vi "Curtin_DAQ.vi"(11 "Settings":T1={"Name of test"="SoundCard--NI 01", "Date"=timestamp(0 s since 1904-01-01), "Location"="Home", "Template"="ScratchPad", "Soundcard"="OCTA-CAPTURE", "resolution"=32, "Sampling rate"=48000, "Ch1 Gain "=1.0, "Ch2 Gain"=1.0, "Sample time (s)"=0.3, "Pre-trigger (s)"=0.001, "Hammer Threshold"=10.0, "Positions"=7, "Taps/Position"=5, "Set Names"="H", "Freq resolution"=1.0, "Hammer cutoff"=0.025, "Mic cutoff"=0.25, "Double bounce "=10.0, "Hammer Cal"=1.0, "dB Offset"=0.0, "Accel Cal"=1.0, "Vibrometer Cal"=1.0, "Mic Cal"=1.0, "Output"=2, "Voltage Cal"=1.0, "Vibrometer Port"="ASRL27::INSTR", "Range"=10, "High Pass"=2, "Bandwidth"=10, "X Range"=[], "Y Range"=[], "dB Spread"=40.0, "Trigger"=0, "Ch_1"=1, "Ch_2"=1, "flip?"=FALSE, "60Hz"=FALSE, "Time offset"=0.0, "Piezo Cal"=1.0, "Default Notes"=""} {"Ch_2" min=1 step=1; "Ch_1" min=1 max=100 step=1; "Trigger" items=["Hammer (force)", "Self-tap", "Spacebar"]; "Bandwidth" items=["1 kHz"=1, "5 kHz"=5, "10 kHz"=10, "25 kHz"=25, "50 kHz"=50, "100 kHz"=100]; "High Pass" items=["Off", "13 Hz", "104 Hz"]; "Range" items=["10 mm/s"=1, "20 mm/s"=2, "50 mm/s"=5, "100 mm/s"=10, "200 mm/s"=20, "500 mm/s"=50, "1 m/s"=100, "2 m/s"=200]; "Output" items=["Accelerometer", "Speed (from acceleration)", "Microphone", "Vibrometer", "Piezo"]; "Voltage Cal" format="%#_13g"; "Ch2 Gain" format="%#_13g"; "Ch1 Gain" format="%#_13g"; "Double bounce" min=0.0; "Mic cutoff" min=0.0 format="%#_4g"; "Hammer cutoff" min=0.0 format="%#_4g"; "Freq resolution" min=0.0; "Pre-trigger (s)" format="%#_13g"; "Date" format="%<%H:%M\n%d/%m/%y>T"; "resolution" items=["16 bit"=16, "24 bit"=24, "32 bit"=32]; "Sampling rate" items=["22050 samp/s"=22050, "44100 samp/s"=44100, "48000 samp/s"=48000]}) -> (3 "Settings out":T1={"Name of test"="SoundCard--NI 01", "Date"=timestamp(0 s since 1904-01-01), "Location"="Home", "Template"="ScratchPad", "Soundcard"="OCTA-CAPTURE", "resolution"=32, "Sampling rate"=48000, "Ch1 Gain "=1.0, "Ch2 Gain"=1.0, "Sample time (s)"=0.3, "Pre-trigger (s)"=0.001, "Hammer Threshold"=10.0, "Positions"=7, "Taps/Position"=5, "Set Names"="H", "Freq resolution"=1.0, "Hammer cutoff"=0.025, "Mic cutoff"=0.25, "Double bounce "=10.0, "Hammer Cal"=1.0, "dB Offset"=0.0, "Accel Cal"=1.0, "Vibrometer Cal"=1.0, "Mic Cal"=1.0, "Output"=2, "Voltage Cal"=1.0, "Vibrometer Port"="ASRL27::INSTR", "Range"=10, "High Pass"=2, "Bandwidth"=10, "X Range"=[], "Y Range"=[], "dB Spread"=40.0, "Trigger"=0, "Ch_1"=1, "Ch_2"=1, "flip?"=FALSE, "60Hz"=FALSE, "Time offset"=0.0, "Piezo Cal"=1.0, "Default Notes"=""} {"Ch_2" min=1 step=1; "Ch_1" min=1 max=100 step=1; "Trigger" items=["Hammer (force)", "Self-tap", "Spacebar"]; "Bandwidth" items=["1 kHz"=1, "5 kHz"=5, "10 kHz"=10, "25 kHz"=25, "50 kHz"=50, "100 kHz"=100]; "High Pass" items=["Off", "13 Hz", "104 Hz"]; "Range" items=["10 mm/s"=1, "20 mm/s"=2, "50 mm/s"=5, "100 mm/s"=10, "200 mm/s"=20, "500 mm/s"=50, "1 m/s"=100, "2 m/s"=200]; "Output" items=["Accelerometer", "Speed (from acceleration)", "Microphone", "Vibrometer", "Piezo"]; "Voltage Cal" format="%#_13g"; "Ch2 Gain" format="%#_13g"; "Ch1 Gain" format="%#_13g"; "Double bounce" min=0.0; "Mic cutoff" min=0.0 format="%#_4g"; "Hammer cutoff" min=0.0 format="%#_4g"; "Freq resolution" min=0.0; "Pre-trigger (s)" format="%#_13g"; "Date" format="%<%H:%M\n%d/%m/%y>T"; "resolution" items=["16 bit"=16, "24 bit"=24, "32 bit"=32]; "Sampling rate" items=["22050 samp/s"=22050, "44100 samp/s"=44100, "48000 samp/s"=48000]})   [LabVIEW 2022 SP3]
doc: "This example demonstrates how to continuously acquire buffered acceleration, sound pressure, or force measurements from IEPE sensors using a DAQmx device.\n\nFor instructions on how to connect your signals to the DAQ device, refer to your device documentation."
uses:
  <vilib>/Utility/error.llb/DialogType.ctl
  ViolinSubs/Mic/Mic_Global.vi
  <vilib>/Utility/miscctls.llb/LVRectTypeDef.ctl
  <vilib>/Waveform/WDTOps.llb/WDT Append Waveforms DBL.vi
  <vilib>/DAQmx/read.llb/DAQmx Read (Analog 1D Wfm NChan NSamp).vi
  ViolinSubs/PreferencesControl.ctl
panel:
  out "Sensitivity (V/X)":dbl[](array[numeric])
  in  "Reset":bool
  in  "Test":bool
  in  "Params":T2={"Sample Clock Source"="OnboardClock", "Sample Rate"=48000, "Hammer"={"Physical Channel"="Dev2/ai0", "Terminal Configuration"=12529, "IEPE Source"=10200, "Current (A)"=0.004, "Trigger"=0, "Min Force"=-100.0, "Max Force"=100.0, "Force Sensitivity (mV/N)"=50.0}, "Microphone"={"Physical Channel"="Dev2/ai1", "Terminal Configuration"=12529, "IEPE Source"=10200, "Current (A)"=0.004, "Output"=2, "Min SPL/Acc"=0.0, "Max SPL/Acc"=120.0, "Sensitivity (mV/g or mV/Pa)"=10.0}} {"Microphone"."Output" items=["Accelerometer", "Accel (speed)", "Microphone", "Vibrometer"]; "Microphone"."IEPE Source" items=["Internal"=10200, "External"=10167, "None"=10230]; "Microphone"."Terminal Configuration" items=["default"=-1, "RSE"=10083, "NRSE"=10078, "Differential"=10106, "Pseudodifferential"=12529]; "Hammer"."Trigger" items=["Hammer (force)", "Self-tap"]; "Hammer"."IEPE Source" items=["Internal"=10200, "External"=10167, "None"=10230]; "Hammer"."Terminal Configuration" items=["default"=-1, "RSE"=10083, "NRSE"=10078, "Differential"=10106, "Pseudodifferential"=12529]}
  in  "Save Settings":bool
  out "Full":bool
  in  "Tab Control":T3(tab)
  out "data":waveform(dbl)[](graph)
  out "Hammer Spectra":cluster{dbl, "df":dbl, "FFT {X}":dbl[]}[](graph)
  out "Microphone Spectra":cluster{"x0":dbl, "df":dbl, dbl[]}[](graph)
  out "Hammer":cluster{dbl, "df":dbl, "FFT {X}":dbl[]}[](graph)
  out "Mic plot":cluster{"x0":dbl, "df":dbl, dbl[]}[](graph)
  in  "Sample time (s)":dbl=0.01 format="%#_13g"
  in  "Method":enum16{"Sqrt(H1H2)", "H1", "H2"}(ring)=enum."H1"
  in  "Pre-trigger (s)":dbl=0.01 format="%#_13g"
  out "Actual Sample Rate":dbl format="%0.2f"
  out "Samples per Loop":i32=300
  in  "View":u16(ring)=2 items=["Raw", "Volts", "Units (Pa, N, mm/s etc)"]
  in  "Threshold (V)":dbl(slide)=0.2 scale=0.0..1.0
  out "live":waveform(dbl)[](graph)
  out "FRF":cluster{dbl, "df":dbl, dbl[]}[](graph)
  # "DAQ Setup"
  # "Live data"
  # "Hz"
  # "dB"
  # "dB"
  # "sec"
  # "sec"
  # "mV/Pa"
  # "mV/m/s2"
  # "mV/mm/s"
  # "V/N"
  # "sec"
  # "sec"
  # "mV/N"
  # "a.u."
  # "a.u."
  # "sec"
  # "Timing Settings"
  # "Hz"
  # "dB"
  # "dB"
  # "sec"
  # "sec"
  # "mV/Pa"
  # "mV/m/s2"
  # "mV/mm/s"
  # "V/N"
  # "sec"
  # "sec"
  # "mV/N"
  # "a.u."
  # "a.u."
  # "sec"
  # "Triggered Data"
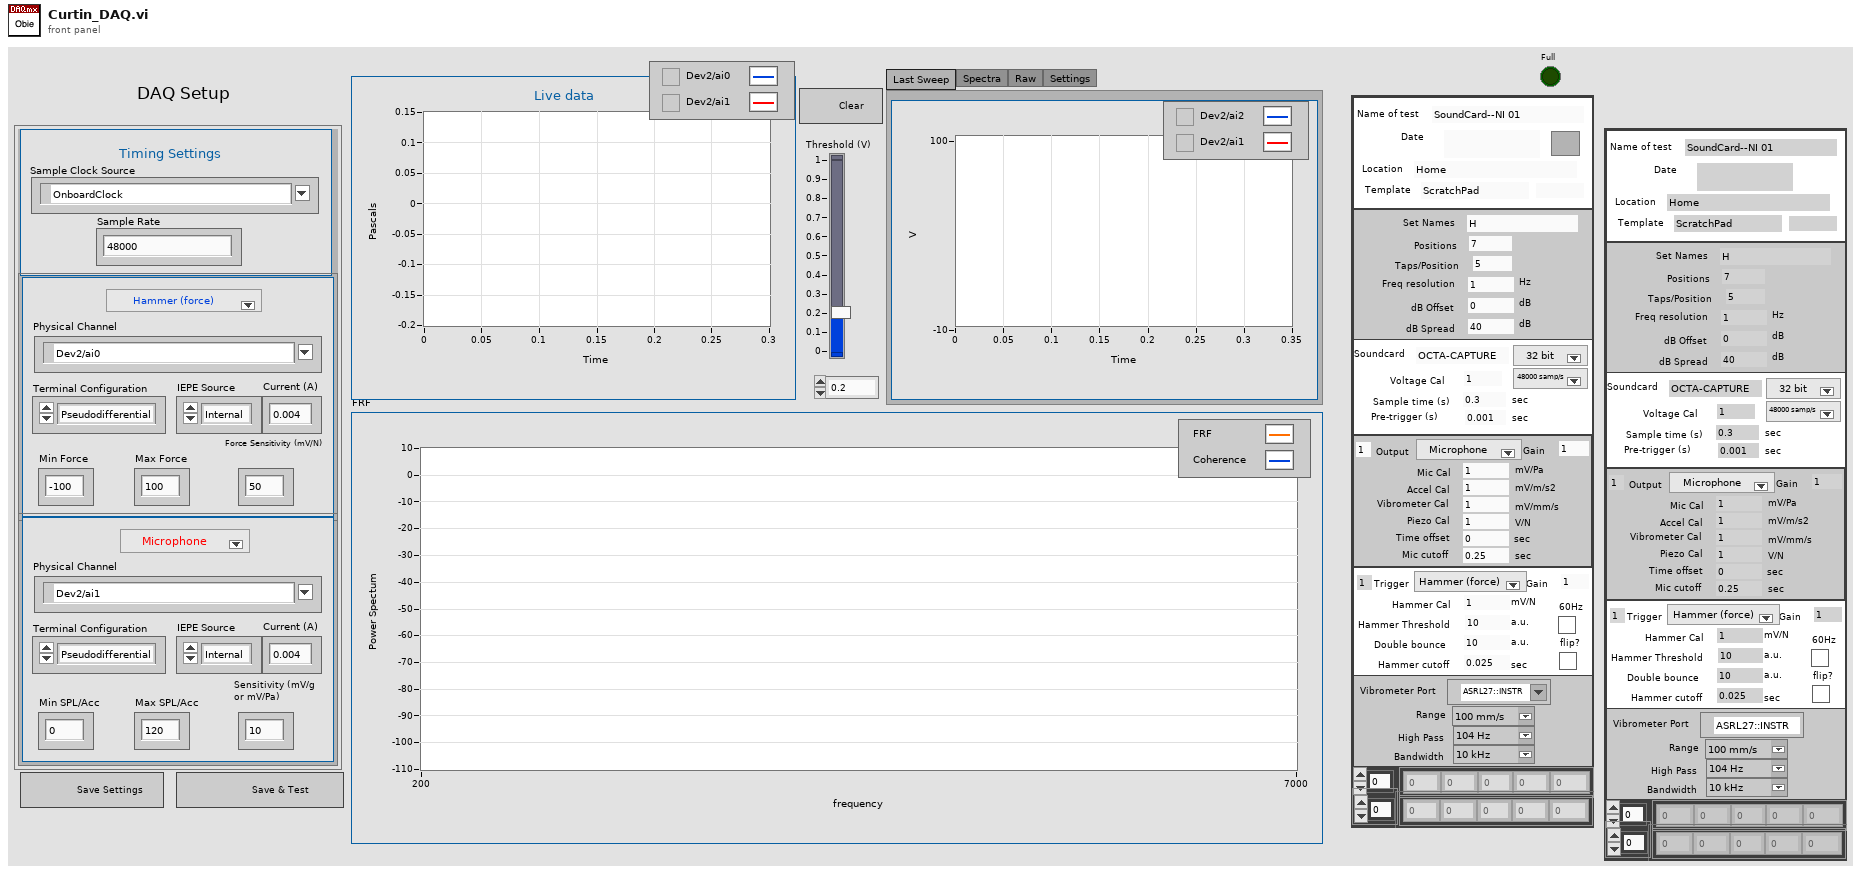
[diagram p1: front panel]
types:
  T1 = typedef "PreferencesControl.ctl" = cluster{"Name of test":string, "Date":timestamp, "Location":string, "Template":string, "Soundcard":string, "resolution":u16, "Sampling rate":u16, "Ch1 Gain ":dbl, "Ch2 Gain":dbl, "Sample time (s)":dbl, "Pre-trigger (s)":dbl, "Hammer Threshold":dbl, "Positions":i16, "Taps/Position":i16, "Set Names":string, "Freq resolution":dbl, "Hammer cutoff":dbl, "Mic cutoff":dbl, "Double bounce ":dbl, "Hammer Cal":dbl, "dB Offset":dbl, "Accel Cal":dbl, "Vibrometer Cal":dbl, "Mic Cal":dbl, "Output":u16, "Voltage Cal":dbl, "Vibrometer Port":refnum<visa-resource-name>, "Range":u16, "High Pass":u16, "Bandwidth":u16, "X Range":cluster{"Minimum":dbl, "Maximum":dbl, "Increment":dbl, "Minor Increment":dbl, "Start":dbl}[], "Y Range":cluster{"Minimum":dbl, "Maximum":dbl, "Increment":dbl, "Minor Increment":dbl, "Start":dbl}[], "dB Spread":dbl, "Trigger":u16, "Ch_1":u8, "Ch_2":u8, "flip?":bool, "60Hz":bool, "Time offset":dbl, "Piezo Cal":dbl, "Default Notes":string}
  T2 = cluster{"Sample Clock Source":tag, "Sample Rate":u32, "Hammer":cluster{"Physical Channel":tag, "Terminal Configuration":i32, "IEPE Source":i32, "Current (A)":dbl, "Trigger":u16, "Min Force":dbl, "Max Force":dbl, "Force Sensitivity (mV/N)":dbl}, "Microphone":cluster{"Physical Channel":tag, "Terminal Configuration":i32, "IEPE Source":i32, "Current (A)":dbl, "Output":u16, "Min SPL/Acc":dbl, "Max SPL/Acc":dbl, "Sensitivity (mV/g or mV/Pa)":dbl}}
  T3 = enum32{"Last Sweep", "Spectra", "Raw", "Settings"}
  T4 = typedef "LVRectTypeDef.ctl" = cluster{"Left":i16, "Top":i16, "Right":i16, "Bottom":i16}
  T5 = cluster{"Alerts":bool, "Log X Axis":bool, "dB scale":bool, "Averaging":bool, "Fade":dbl, "Centroids?":bool}
  T6 = cluster{"Physical Channel":tag, "Terminal Configuration":i32, "IEPE Source":i32, "Current (A)":dbl, "Trigger":u16, "Min Force":dbl, "Max Force":dbl, "Force Sensitivity (mV/N)":dbl}
  T7 = cluster{"Physical Channel":tag, "Terminal Configuration":i32, "IEPE Source":i32, "Current (A)":dbl, "Output":u16, "Min SPL/Acc":dbl, "Max SPL/Acc":dbl, "Sensitivity (mV/g or mV/Pa)":dbl}
  T8 = typedef "DialogType.ctl" = u16
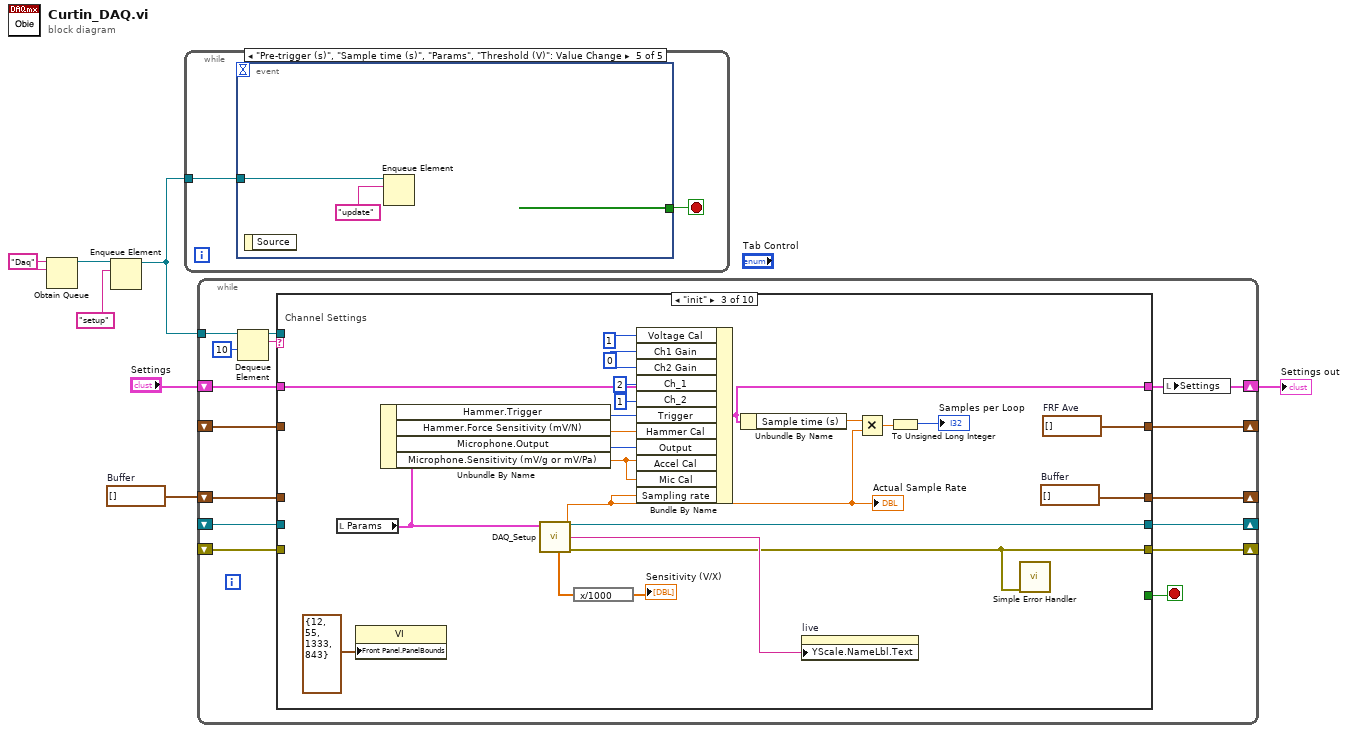
[diagram p0: block diagram]
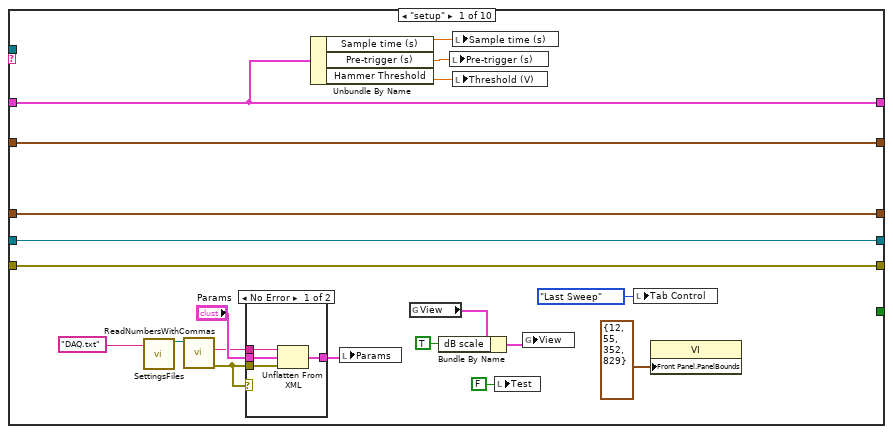
[diagram p2: hidden frame]
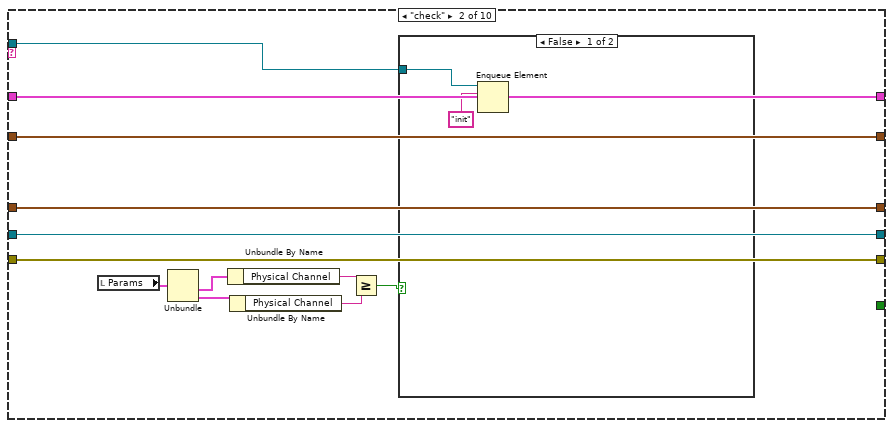
[diagram p4: hidden frame]
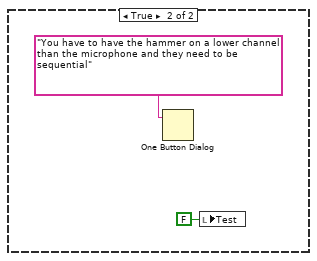
[diagram p5: hidden frame]
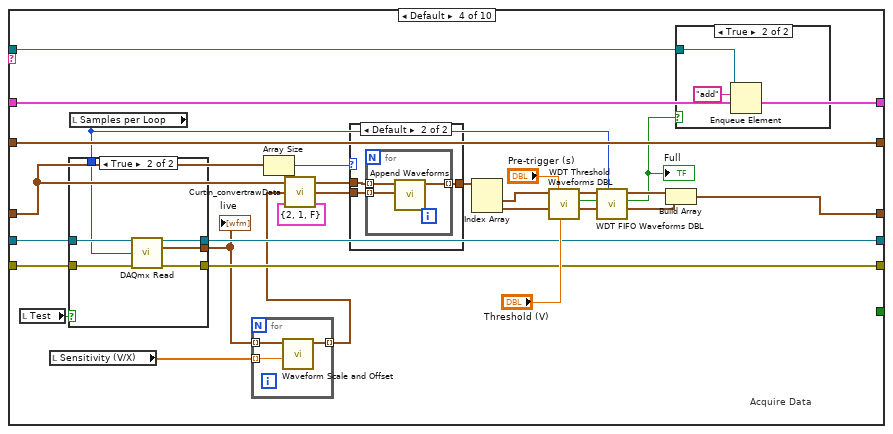
[diagram p6: hidden frame]
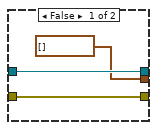
[diagram p7: hidden frame]
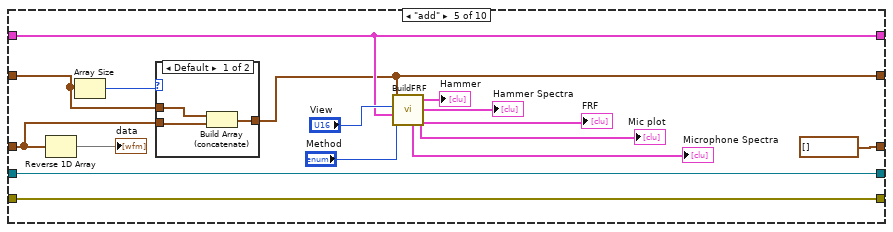
[diagram p10: hidden frame]
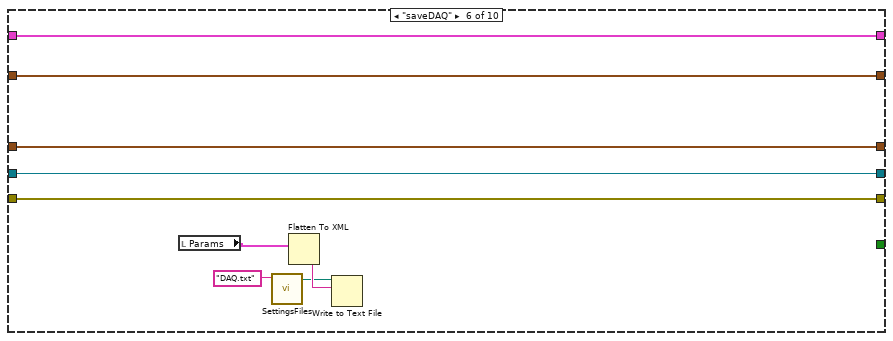
[diagram p12: hidden frame]
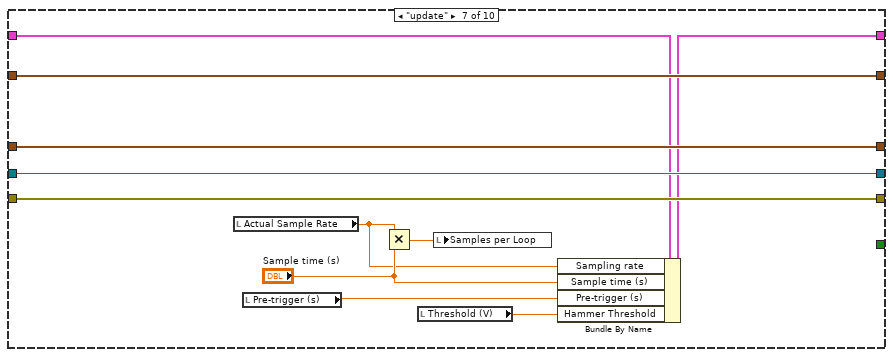
[diagram p13: hidden frame]
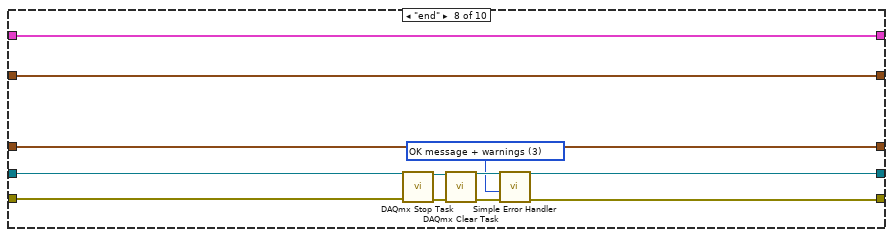
[diagram p14: hidden frame]
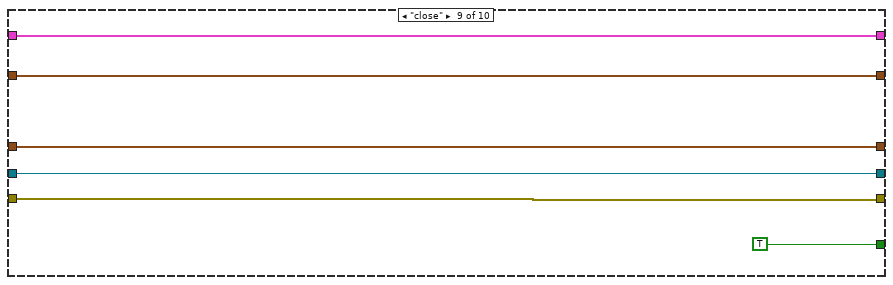
[diagram p15: hidden frame]
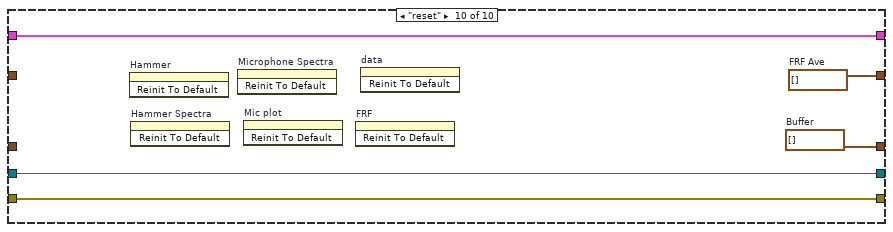
[diagram p16: hidden frame]
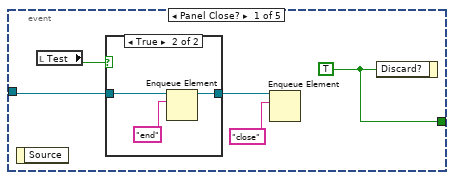
[diagram p17: hidden frame]
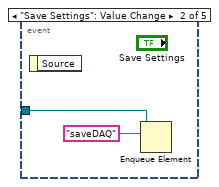
[diagram p19: hidden frame]
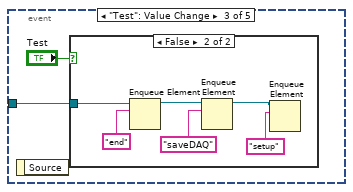
[diagram p20: hidden frame]
diagram:
  w5 = "Daq" ("name (unnamed)")
  w6 = waveform(dbl)[] []  # Buffer
  n1 = Obtain Queue(name (unnamed)=w5, element data type=w5) -> (queue out=w4:refnum<queue>)  [unwired: 3 in, 2 out]
  n2 = Enqueue Element(queue=w4, element="setup") -> (queue out=w3:refnum<queue>)  [unwired: 2 in, 2 out]
  n3 = while {
    tunnel: w3 -> [w9]
    stop <- w8 stop-if-true
    n4 = event shown="[4] \"Pre-trigger (s)\", \"Sample time (s)\", \"Params\", \"Threshold (V)\": Value Change" {
      selector: _ -> [_ _ _ _ _]
      dyn-events: _ -> [_ _ _ _ _]
      timeout: _ -> [_ _ _ _ _]
      tunnel: w9 -> [w14 w20 w22 w34 w36]
      tunnel: [w13 _ _ _ _] -> w8
      event Panel Close? {
        w13 = TRUE ("Discard?")
        n5 = event-data() -> ()  [unwired: 1 in, 1 out]
        n6 = local read "Test"() -> (w10:bool)
        n7 = case shown="True" w10 {
          tunnel: w14 -> [w15 w18]
          tunnel: [w15 w16] -> w11
          frame False {
          }
          frame True {
            n8 = Enqueue Element(queue=w18, element="end") -> (queue out=w16:refnum<queue>)  [unwired: 2 in, 2 out]
          }
        }
        n9 = Enqueue Element(queue=w11, element="close") -> ()  [unwired: 2 in, 3 out]
        n10 = event-data("Discard?"=w13) -> ()  [unwired: 1 in, 1 out]
      }
      event "Save Settings": Value Change {
        n11 = event-data() -> ()  [unwired: 1 in, 1 out]
        n12 = Enqueue Element(queue=w20, element="saveDAQ") -> ()  [unwired: 2 in, 3 out]
      }
      event "Test": Value Change {
        n13 = event-data() -> ()  [unwired: 1 in, 1 out]
        n14 = case shown="False" "Test" {
          tunnel: w22 -> [w26 w30]
          frame True {
            n15 = Enqueue Element(queue=w26, element="saveDAQ") -> (queue out=w23:refnum<queue>)  [unwired: 2 in, 2 out]
            n16 = Enqueue Element(queue=w23, element="check") -> ()  [unwired: 2 in, 3 out]
          }
          frame False {
            n17 = Enqueue Element(queue=w30, element="end") -> (queue out=w29:refnum<queue>)  [unwired: 2 in, 2 out]
            n18 = Enqueue Element(queue=w29, element="saveDAQ") -> (queue out=w27:refnum<queue>)  [unwired: 2 in, 2 out]
            n19 = Enqueue Element(queue=w27, element="setup") -> ()  [unwired: 2 in, 3 out]
          }
        }
      }
      event "Reset": Value Change {
        n20 = event-data() -> ()  [unwired: 1 in, 1 out]
        n21 = Enqueue Element(queue=w34, element="reset") -> ()  [unwired: 2 in, 3 out]
      }
      event "Pre-trigger (s)", "Sample time (s)", "Params", "Threshold (V)": Value Change {
        n22 = event-data() -> ()  [unwired: 1 in, 1 out]
        n23 = Enqueue Element(queue=w36, element="update") -> ()  [unwired: 2 in, 3 out]
      }
    }
  }
  n24 = while {
    tunnel: w3 -> [w50]
    shift-right: [w49] -> _
    shift-left: _ -> [w48]
    shift-right: [w42] -> w1
    shift-left: "Settings" -> [w45]
    shift-right: [w37] -> _
    shift-left: w6 -> [w44]
    shift-right: [w46] -> _
    shift-left: _ -> [w47]
    shift-right: [w40] -> _
    shift-left: _ -> [w43]
    stop <- w41 stop-if-true
    n25 = Dequeue Element(queue=w50, timeout in ms (-1)=10) -> (queue out=w38:refnum<queue>, element=w51:string)  [unwired: 1 in, 2 out]
    n26 = case shown="\"init\"" w51 {
      tunnel: [w65 w85 w115 w129 w167 w191 w203 w210 w216 w225] -> w49
      tunnel: w48 -> [w65 w85 _ w132 w167 w191 w203 w213 w216 w225]
      tunnel: [w60 w88 w104 w128 w168 w193 w196 w214 w220 w224] -> w42
      tunnel: [w66 w86 w114 w133 waveform(dbl)[] [] w192 w204 w209 w219 w221] -> w37
      tunnel: w47 -> [w64 w84 _ w131 w166 w190 w202 w212 w215 w223]
      tunnel: [w64 w84 w106 w130 w166 w190 w202 w211 w215 w223] -> w46
      tunnel: w45 -> [w60 w88 w108 w128 w168 w193 w195 w214 w220 w224]
      tunnel: w44 -> [w66 w86 _ w127 w180 w192 w204 w209 w219 _]
      tunnel: w43 -> [w63 w87 _ w126 w178 w187 w201 w208 w217 _]
      tunnel: [_ _ _ _ _ _ _ _ TRUE _] -> w41
      tunnel: [w63 w87 w113 w126 w165 w187 w201 w208 w217 w222] -> w40
      tunnel: w38 -> [_ w81 _ w125 _ _ _ _ _ _]
      frame "setup" {
        n27 = call "SettingsFiles.vi"("settings file name"="DAQ.txt" ("name or relative path")) -> ("file path"=w52:path)  [unwired: 9 in, 1 out]
        n28 = call "ReadNumbersWithCommas.vi"("file (use dialog)"=w52) -> ("error out"=w54:errorcluster, "text"=w55:string)  [unwired: 7 in, 2 out]
        n29 = case shown="No Error" w54 {
          tunnel: w55 -> [w75 _]
          tunnel: w54 -> [w74 _]
          tunnel: "Params" -> [w73 w76]
          tunnel: [w72 w76] -> w70
          frame No Error {
            n30 = Unflatten From XML(xml string=w75, type=w73, error in (no error)=w74) -> (value=w72:T2)  [unwired: 1 out]
          }
          frame Error {
          }
        }
        n31 = Unbundle By Name(w60) -> ("Sample time (s)"=w58:dbl, "Pre-trigger (s)"=w59:dbl, "Hammer Threshold"=w56:dbl)
        n32 = local write "Params"(w70) -> ()
        n33 = global read "Mic_Global.vi" "View"() -> (w68:T5)
        n34 = Bundle By Name(cluster=w68, "dB scale"=TRUE) -> (w69:T5)
        n35 = local write "Pre-trigger (s)"(w59) -> ()
        n36 = local write "Sample time (s)"(w58) -> ()
        n37 = local write "Threshold (V)"(w56) -> ()
        n38 = local write "Test"(FALSE ("Test")) -> ()
        n39 = global write "Mic_Global.vi" "View"(w69) -> ()
        n40 = local write "Tab Control"(T3."Last Sweep" ("Tab Control")) -> ()
        n41 = property class="VI"("Front Panel.PanelBounds"=T4 {"Left"=12, "Top"=55, "Right"=352, "Bottom"=829} ("Front Panel Window:Panel Bounds")) -> ()  [unwired: 2 in, 2 out]
      }
      frame "check" {
        n42 = local read "Params"() -> (w83:T2)
        n43 = Unbundle(w83) -> ("Hammer"=w80:T6, "Microphone"=w79:T7)  [unwired: 2 out]
        n44 = Unbundle By Name(w80) -> ("Physical Channel"=w78:tag)
        n45 = Unbundle By Name(w79) -> ("Physical Channel"=w77:tag)
        n46 = Greater Or Equal?(x=w78, y=w77) -> (x >= y?=w82:bool)
        n47 = case shown="False" w82 {
          tunnel: w81 -> [w89 _]
          frame False {
            n48 = Enqueue Element(queue=w89, element="init") -> ()  [unwired: 2 in, 3 out]
          }
          frame True {
            n49 = One Button Dialog(message="You have to have the hammer on a lower channel than the microphone and they need to be sequential") -> ()  [unwired: 1 in, 1 out]
            n50 = local write "Test"(FALSE ("Test")) -> ()
          }
        }
      }
      frame "init" {
        w96 = u8 0 ("Ch_1")
        w113 = waveform(dbl)[] []  # FRF Ave
        w114 = waveform(dbl)[] []  # Buffer
        # "Channel Settings"
        n51 = local read "Params"() -> (w103:T2)
        n52 = property class="VI"("Front Panel.PanelBounds"=T4 {"Left"=12, "Top"=55, "Right"=1333, "Bottom"=843} ("Front Panel Window:Panel Bounds")) -> ()  [unwired: 2 in, 2 out]
        n53 = Unbundle By Name(w103) -> ("Hammer.Trigger"=w102:u16, "Hammer.Force Sensitivity (mV/N)"=w101:dbl, "Microphone.Output"=w100:u16, "Microphone.Sensitivity (mV/g or mV/Pa)"=w99:dbl)
        n54 = call "DAQ_Setup.vi"("Params"=w103) -> ("error out"=w106:errorcluster, "SampClk.Rate"=w105:dbl, "Y axis Label"=w111:string, "Task out"=w115:refnum<k21>, "Sensitivity (mV/X)"=w94:dbl[])  [unwired: 6 in]
        "Actual Sample Rate" <- w105
        n55 = expression code="x/1000"(w94) -> (→"Sensitivity (V/X)":dbl[])
        n56 = Bundle By Name(cluster=w108, "Voltage Cal"=u8 1 ("Ch_1"), "Ch1 Gain"=w96, "Ch2 Gain"=w96, "Ch_1"=u8 2, "Ch_2"=u8 1, "Trigger"=w102, "Hammer Cal"=w101, "Output"=w100, "Accel Cal"=w99, "Mic Cal"=w99, "Sampling rate"=w105) -> (w104:T1)
        n57 = Unbundle By Name(w104) -> ("Sample time (s)"=w110:dbl)
        n58 = property on="live" class="WFGraph (strict)"("YScale.NameLbl.Text"=w111) -> ()  [unwired: 2 in, 2 out]
        n59 = Multiply(x=w110, y=w105) -> (x*y=w109:dbl)
        n60 = To Unsigned Long Integer(number=w109) -> (unsigned 32bit integer=→"Samples per Loop":u32)
        n61 = call <vilib>:"Simple Error Handler.vi"("error in (no error)"=w106) -> ()  [unwired: 4 in, 5 out]
      }
      frame Default {
        # "Acquire Data"
        n62 = local read "Test"() -> (w122:bool)
        n63 = local read "Sensitivity (V/X)"() -> (w116:dbl[])
        n64 = local read "Samples per Loop"() -> (w121:i32)
        n65 = case shown="True" w122 {
          tunnel: [waveform(dbl)[] [] ("data") w155] -> w117
          tunnel: w132 -> [w149 w154]
          tunnel: w131 -> [w147 w153]
          tunnel: [w147 w152] -> w130
          tunnel: [w149 w151] -> w129
          tunnel: w121 -> [_ w150]
          frame False {
          }
          frame True {
            n66 = call-poly <vilib>:"DAQmx Read.vi"("task/channels in"=w154, "number of samples per channel"=w150, "error in"=w153) -> ("task out"=w151:refnum<k21>, "data"=w155:waveform(dbl)[], "error out"=w152:errorcluster)  [unwired: 10 in]
          }
        }
        "live" <- w117
        n67 = for {
          tunnel: w117 -> [w146] mode=indexing
          tunnel: w116 -> [w145] mode=indexing
          tunnel: [w144] -> w118 mode=indexing
          n68 = call <vilib>:"Waveform Scale and Offset.vi"("scale"=w145, "waveform in"=w146) -> ("waveform out"=w144:waveform(dbl))  [unwired: 8 in, 1 out]
        }
        n69 = Array Size(array=w127) -> (size(s)=w138:i32)
        n70 = call "Curtin_convertrawData.vi"("incoming data"=w118, "Ports"=cluster{"Ch_1":u8, "Ch_2":u8, bool} {"Ch_1"=2, "Ch_2"=1, FALSE}) -> ("Ordered"=w119:waveform(dbl)[])
        n71 = case shown="Default" w138 {
          tunnel: w119 -> [w158 w161]
          tunnel: w127 -> [_ w160]
          tunnel: [w158 w159] -> w137
          frame 0 {
          }
          frame Default {
            n72 = for {
              tunnel: w161 -> [w164] mode=indexing
              tunnel: [w163] -> w159 mode=indexing
              tunnel: w160 -> [w162] mode=indexing
              n73 = call-poly <vilib>:"Append Waveforms.vi"("waveform B"=w164, "waveform A"=w162) -> ("waveform out"=w163:waveform(dbl))  [unwired: 8 in, 1 out]
            }
          }
        }
        n74 = Index Array(array=w137) -> (element #1=w123:waveform(dbl), element #2=w140:waveform(dbl))  [unwired: 2 in]
        n75 = call "WDT Threshold Waveforms DBL.vi"("A Threshold"="Threshold (V)", "Pre-trigger (s)"="Pre-trigger (s)", "Hammer"=w140, "Mic"=w123) -> ("Hammer out"=w134:waveform(dbl), "Triggered?"=w136:bool, "Mic out"=w135:waveform(dbl))  [unwired: 4 in, 1 out]
        n76 = call "WDT FIFO Waveforms DBL.vi"("FIFO"=w121, "Hammer"=w134, "Triggered?"=w136, "Mic"=w135) -> ("Hammer out"=w143:waveform(dbl), "Full"=w124:bool, "Mic out"=w142:waveform(dbl))  [unwired: 4 in, 1 out]
        "Full" <- w124
        n77 = Build Array(w142, w143) -> (w133:waveform(dbl)[])
        n78 = case shown="True" w124 {
          tunnel: w125 -> [_ w156]
          frame False {
          }
          frame True {
            n79 = Enqueue Element(queue=w156, element="add") -> ()  [unwired: 2 in, 3 out]
          }
        }
      }
      frame "add" {
        n80 = Reverse 1D Array(array=w180) -> (reversed array=→"data":waveform(dbl)[])
        n81 = Array Size(array=w178) -> (size(s)=w177:i32)
        n82 = case shown="Default" w177 {
          tunnel: [w182 w184] -> w165
          tunnel: w178 -> [w183 _]
          tunnel: w180 -> [w181 w184]
          frame Default {
            n83 = Build Array (concatenate)(w183, w181) -> (w182:waveform(dbl)[])
          }
          frame 0 {
          }
        }
        n84 = call "BuildFRF.vi"("Method"="Method", "Settings"=w168, "View"="View", "Data In"=w165) -> ("Average FRF"=→"FRF":cluster{dbl, "df":dbl, dbl[]}[], "Microphone"=→"Mic plot":cluster{dbl, "dt":dbl, "Y":dbl[]}[], "Hammer"=→"Hammer":cluster{dbl, "dt":dbl, "Y":dbl[]}[], "Microphone Spectra"=→"Microphone Spectra":cluster{"x0":dbl, "df":dbl, dbl[]}[], "Hammer Spectra"=→"Hammer Spectra":cluster{dbl, "df":dbl, "FFT {X}":dbl[]}[])  [unwired: 2 in, 1 out]
      }
      frame "saveDAQ" {
        n85 = local read "Params"() -> (w188:T2)
        n86 = call "SettingsFiles.vi"("settings file name"="DAQ.txt" ("name or relative path")) -> ("file path"=w185:path)  [unwired: 9 in, 1 out]
        n87 = Flatten To XML(6:w188) -> (2:w189:string)
        n88 = Write to Text File(file (use dialog)=w185, text=w189) -> ()  [unwired: 2 in, 3 out]
      }
      frame "update" {
        n89 = local read "Actual Sample Rate"() -> (w197:dbl)
        n90 = local read "Pre-trigger (s)"() -> (w199:dbl)
        n91 = Multiply(x=w197, y="Sample time (s)") -> (x*y=w200:dbl)
        n92 = local read "Threshold (V)"() -> (w194:dbl)
        n93 = local write "Samples per Loop"(w200) -> ()
        n94 = Bundle By Name(cluster=w195, "Sampling rate"=w197, "Sample time (s)"="Sample time (s)", "Pre-trigger (s)"=w199, "Hammer Threshold"=w194) -> (w196:T1)
      }
      frame "end" {
        w205 = T8 3 items=["no dialog", "OK message", "continue or stop message", "OK message + warnings", "continue/stop + warnings"] ("type of dialog (OK msg:1)")
        n95 = call <vilib>:"DAQmx Stop Task.vi"("task/channels in"=w213, "error in"=w212) -> ("task out"=w210:refnum<k21>, "error out"=w207:errorcluster)  [unwired: 12 in]
        n96 = call <vilib>:"DAQmx Clear Task.vi"("task in"=w210, "error in"=w207) -> ("error out"=w206:errorcluster)  [unwired: 13 in]
        n97 = call <vilib>:"Simple Error Handler.vi"("type of dialog (OK msg:1)"=w205, "error in (no error)"=w206) -> ("error out"=w211:errorcluster)  [unwired: 3 in, 4 out]
      }
      frame "close" {
      }
      frame "reset" {
        w222 = waveform(dbl)[] []  # FRF Ave
        w221 = waveform(dbl)[] []  # Buffer
        n98 = invoke on="Hammer" class="WFGraph (strict)" method="Reinit To Default"() -> ()  [unwired: 3 in, 3 out]
        n99 = invoke on="Hammer Spectra" class="WFGraph (strict)" method="Reinit To Default"() -> ()  [unwired: 3 in, 3 out]
        n100 = invoke on="Microphone Spectra" class="WFGraph (strict)" method="Reinit To Default"() -> ()  [unwired: 3 in, 3 out]
        n101 = invoke on="Mic plot" class="WFGraph (strict)" method="Reinit To Default"() -> ()  [unwired: 3 in, 3 out]
        n102 = invoke on="FRF" class="WFGraph (strict)" method="Reinit To Default"() -> ()  [unwired: 3 in, 3 out]
        n103 = invoke on="data" class="WFGraph (strict)" method="Reinit To Default"() -> ()  [unwired: 3 in, 3 out]
      }
    }
    n104 = local write "Settings"(w42) -> ()
  }
  "Settings out" <- w1
